vi "Set Lockstep Tolerance.vi"(6 "Tolerance":u64, 7 "Lockstep Group (1)":u8=1, 8 "error in (no error)":errorcluster, 9 "Device Number":string, 10 "Secondary Axis Label":string, 11 "VISA resource name":refnum<visa-resource-name>) -> (0 "error out":errorcluster, 3 "VISA resource name out":refnum<visa-resource-name>)   [LabVIEW 2018, in "Zaber A Series.lvlib"]
doc: "Sets the twist tolerance for one or all secondary axes of a lockstep group. Tolerance is expressed in device position units and is relative to the position of the primary (first) axis of a lockstep group. The tolerance is the maximum deviation from the configured axis offset that will be allowed before trajectories are adjusted to reduce the difference. The default is conservative; be cautious in adjusting this value because mechanical damange to your system may result if the tolerance is set too high.\n\nThe Secondary Axis Label input is a letter that represents the rank within the lockstep group of the axis you want to set the tolerance for. 'b' is the first secondary axis, 'c' is the next one, etc. Leave this input empty to set the same tolerance on all secondary axes.\n\nThis VI does not check in advance for error conditions such as lockstep not being supported on the device or no group numbers being available. It does check the error input and takes no action if an error condition already exists.\n\nThis VI requires that the Initialize VI has been called with the same serial port, and that the device has Firmware version 7.11 or later."
uses:
  Zaber A Series.lvlib
  Private/All Commands.ctl
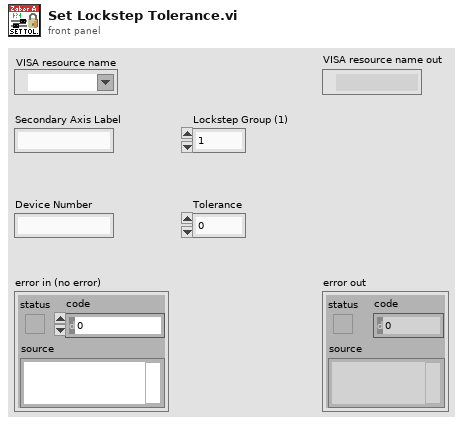
[diagram p1: front panel]
types:
  T1 = typedef "Zaber A Series.lvlib/All Commands.ctl" = string
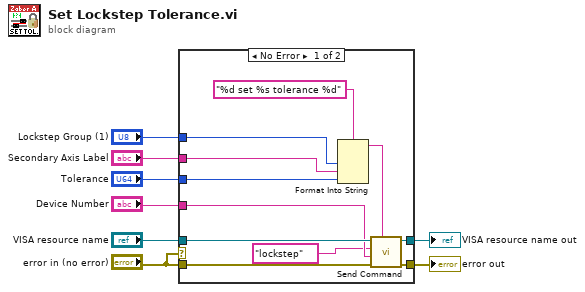
[diagram p0: block diagram]
diagram:
  n1 = case shown="No Error" "error in (no error)" {
    tunnel: "VISA resource name" -> [w19 w21]
    tunnel: [w17 w21] -> w7
    tunnel: [w16 w20] -> w6
    tunnel: "Device Number" -> [w15 _]
    tunnel: "Lockstep Group (1)" -> [w13 _]
    tunnel: "error in (no error)" -> [w11 w20]
    tunnel: "Secondary Axis Label" -> [w10 _]
    tunnel: "Tolerance" -> [w9 _]
    frame No Error {
      n2 = Format Into String(format string="%d set %s tolerance %d", w13, w10, w9) -> (resulting string=w14:string)  [unwired: 2 in, 1 out]
      n3 = call "Send Command.vi"("Data"=w14, "error in (no error)"=w11, "Device and Axis"=w15, "Command"=T1 "lockstep" ("Complete Command List"), "VISA resource name"=w19) -> ("error out"=w16:errorcluster, "VISA resource name out"=w17:refnum<visa-resource-name>)  [unwired: 1 in, 4 out]
    }
    frame Error {
    }
  }
  "VISA resource name out" <- w7
  "error out" <- w6
